vi "CAVRO PUMPS.vi"(0 "Serial Port":refnum<visa-resource-name>="COM3") -> ()   [LabVIEW 2020]
doc: "The Advanced Serial Read and Write example performs a Serial Port Read, a Serial Port Write, or a combination of these actions while setting some advanced serial features like buffer size, termination characters, and XON/XOFF flow control. The user selects the actions (read or write) on the front panel. If both are selected, the VI will write the data first, read the data and then close the VISA session that is opened to the port. \n\nThe parameters set for the serial port must match the parameters of the connected instrument or device. In this example, the bytes to read parameter specifies the number of bytes that the serial port reads. If there were more bytes at the port than the number specified in bytes to read, those bytes would not be read. Also, if you specify to read more bytes than the number of bytes actually read, you might receive a timeout error message.\n\nINSTRUCTIONS:\n1) Select the serial resource and configuration parameters (baud rate, data bits, parity, stop bits, flow control).\n2) Termination character can be enabled and set. Also, set the required input buffer size prior to running the example.\n3) Select the operations to be performed. \n4) Connect the serial port to your device. If no device is available, perform a loopback test by doing one of the following. Short pins 2 and 3 on a RS-232 cable or short pin 4 to pin 8 and pin 5 to pin 9 on a RS-485/422 cable. \n5) Run the VI to see the data read. (The \"read string\" will match the \"string to write\" if a loopback test was performed.)\n\nThis example exposes several advanced features that you may need for your application. Not all applications need all the features shown in this example. The input buffer size is likely an important setting that you want to control in your application. This example expands upon the flow control option for XON and XOFF, allowing the user to choose those control characters. The timeout parameter has been brought to the front panel so a user can specify the time period the VISA Read will wait for the number of bytes to read before timing out. Also, the user has several controls for the termination character, which is discussed later.\n\nNote that you can press the write and read buttons and change the bytes to read parameters on the fly, while the example is running. However, you must stop the example to change the other configuration parameters after the example has started running, and then run again.\n\nSet the I/O buffer size slightly higher the amount of data you expect to receive. This is very important for applications that don't use flow control, as you may lose characters if the receive buffer overflows.\n\nSetting the timeout period ensures that the operation returns with a timeout error if the operation cannot be performed in the specified time period. \n\nSome devices require a termination character in order to identify the end of command strings. Some devices send a termination character to signify the end of data to be read. \n\nThis example shows how you can end the Read operation once a termination character is detected in the buffer and/or append a termination character at the end of the Write data. To enable the Read to end on a termination character, use the VISA Configure Serial Port or use the VISA Properties Serial End Mode for Reads, Termination Character Enable, and Termination Character. To end the Write with a termination character, use the VISA Properties Serial End Mode for Writes, the Send End Enable, and Termination Character. In this example, the same termination character is used for both the Read and the Write. You can specify two different characters for your application, if desired.\n\nYour application may require specific characters for the XON/XOFF Flow Control. You can specify these characters with the VISA Properties Flow Control XOFF Character and Flow Control XON Character. Note that if the standard XON and XOFF characters are used, then decimal 17 and 19 are unavailable for data values. Remember that using flow control and setting an adequate buffer size allow you to prevent buffer overflows."
uses:
  <vilib>/Instr/_visa.llb/VISA Configure Serial Port (Instr).vi
panel:
  in  "Channel":string
  in  "String 3":string
  in  "String 2":string
  in  "String":string="T"
  out "Read buffer":string
  out "Method New/Load":dbl
  in  "WRITE":bool=TRUE
  out "Boolean 2":bool
  out "Boolean":bool
  in  "SLOW SPEED":bool
  in  "FREE COMMAND":bool
  out "String loaded":string caption="String loaded:"
  in  "Load from":path=path "C:/write-read example.txt"
  in  "?":bool
  in  "stop saving":bool
  in  "save":bool
  in  "Save to":path
  in  "INITIALIZE":bool
  in  "END SEQUENCE":bool
  in  "?":string
  in  "DELAY [min]:":bool
  in  "?":string
  in  "GO TO CH:":bool
  in  "INFUSE [uL]:":bool
  out "Command sequence":string
  in  "?":string
  in  "REPEATS & END CICLE":bool
  in  "START CICLE":bool
  in  "REFILL [uL]:":bool
  out "String":string
  in  "START":bool
  # "CAVRO PUMP CONTROLLER"
  # "Load sequence >"
  # "< New sequence"
  # "\"T\" to kill process"
  # "Save to"
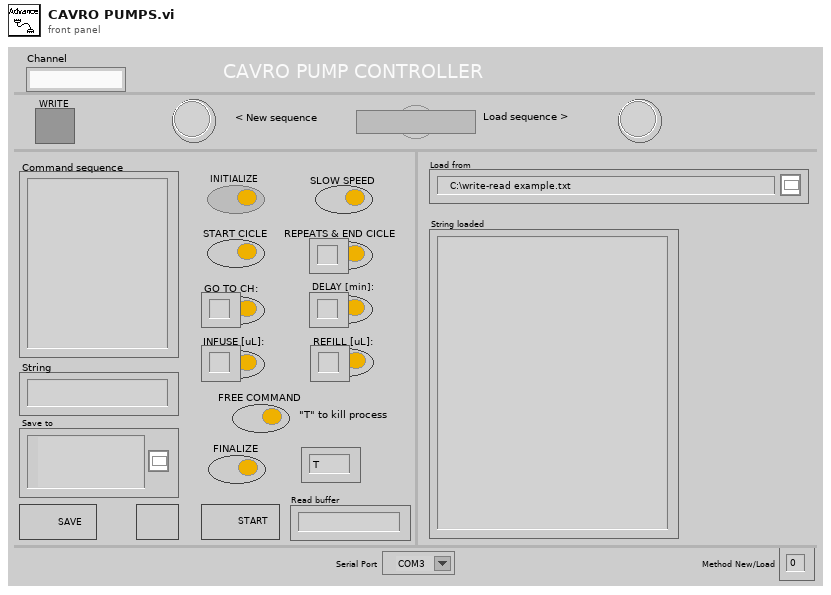
[diagram p1: front panel]
types:
  T1 = enum16{"open", "open or create", "create or replace", "create", "open (read only)"}
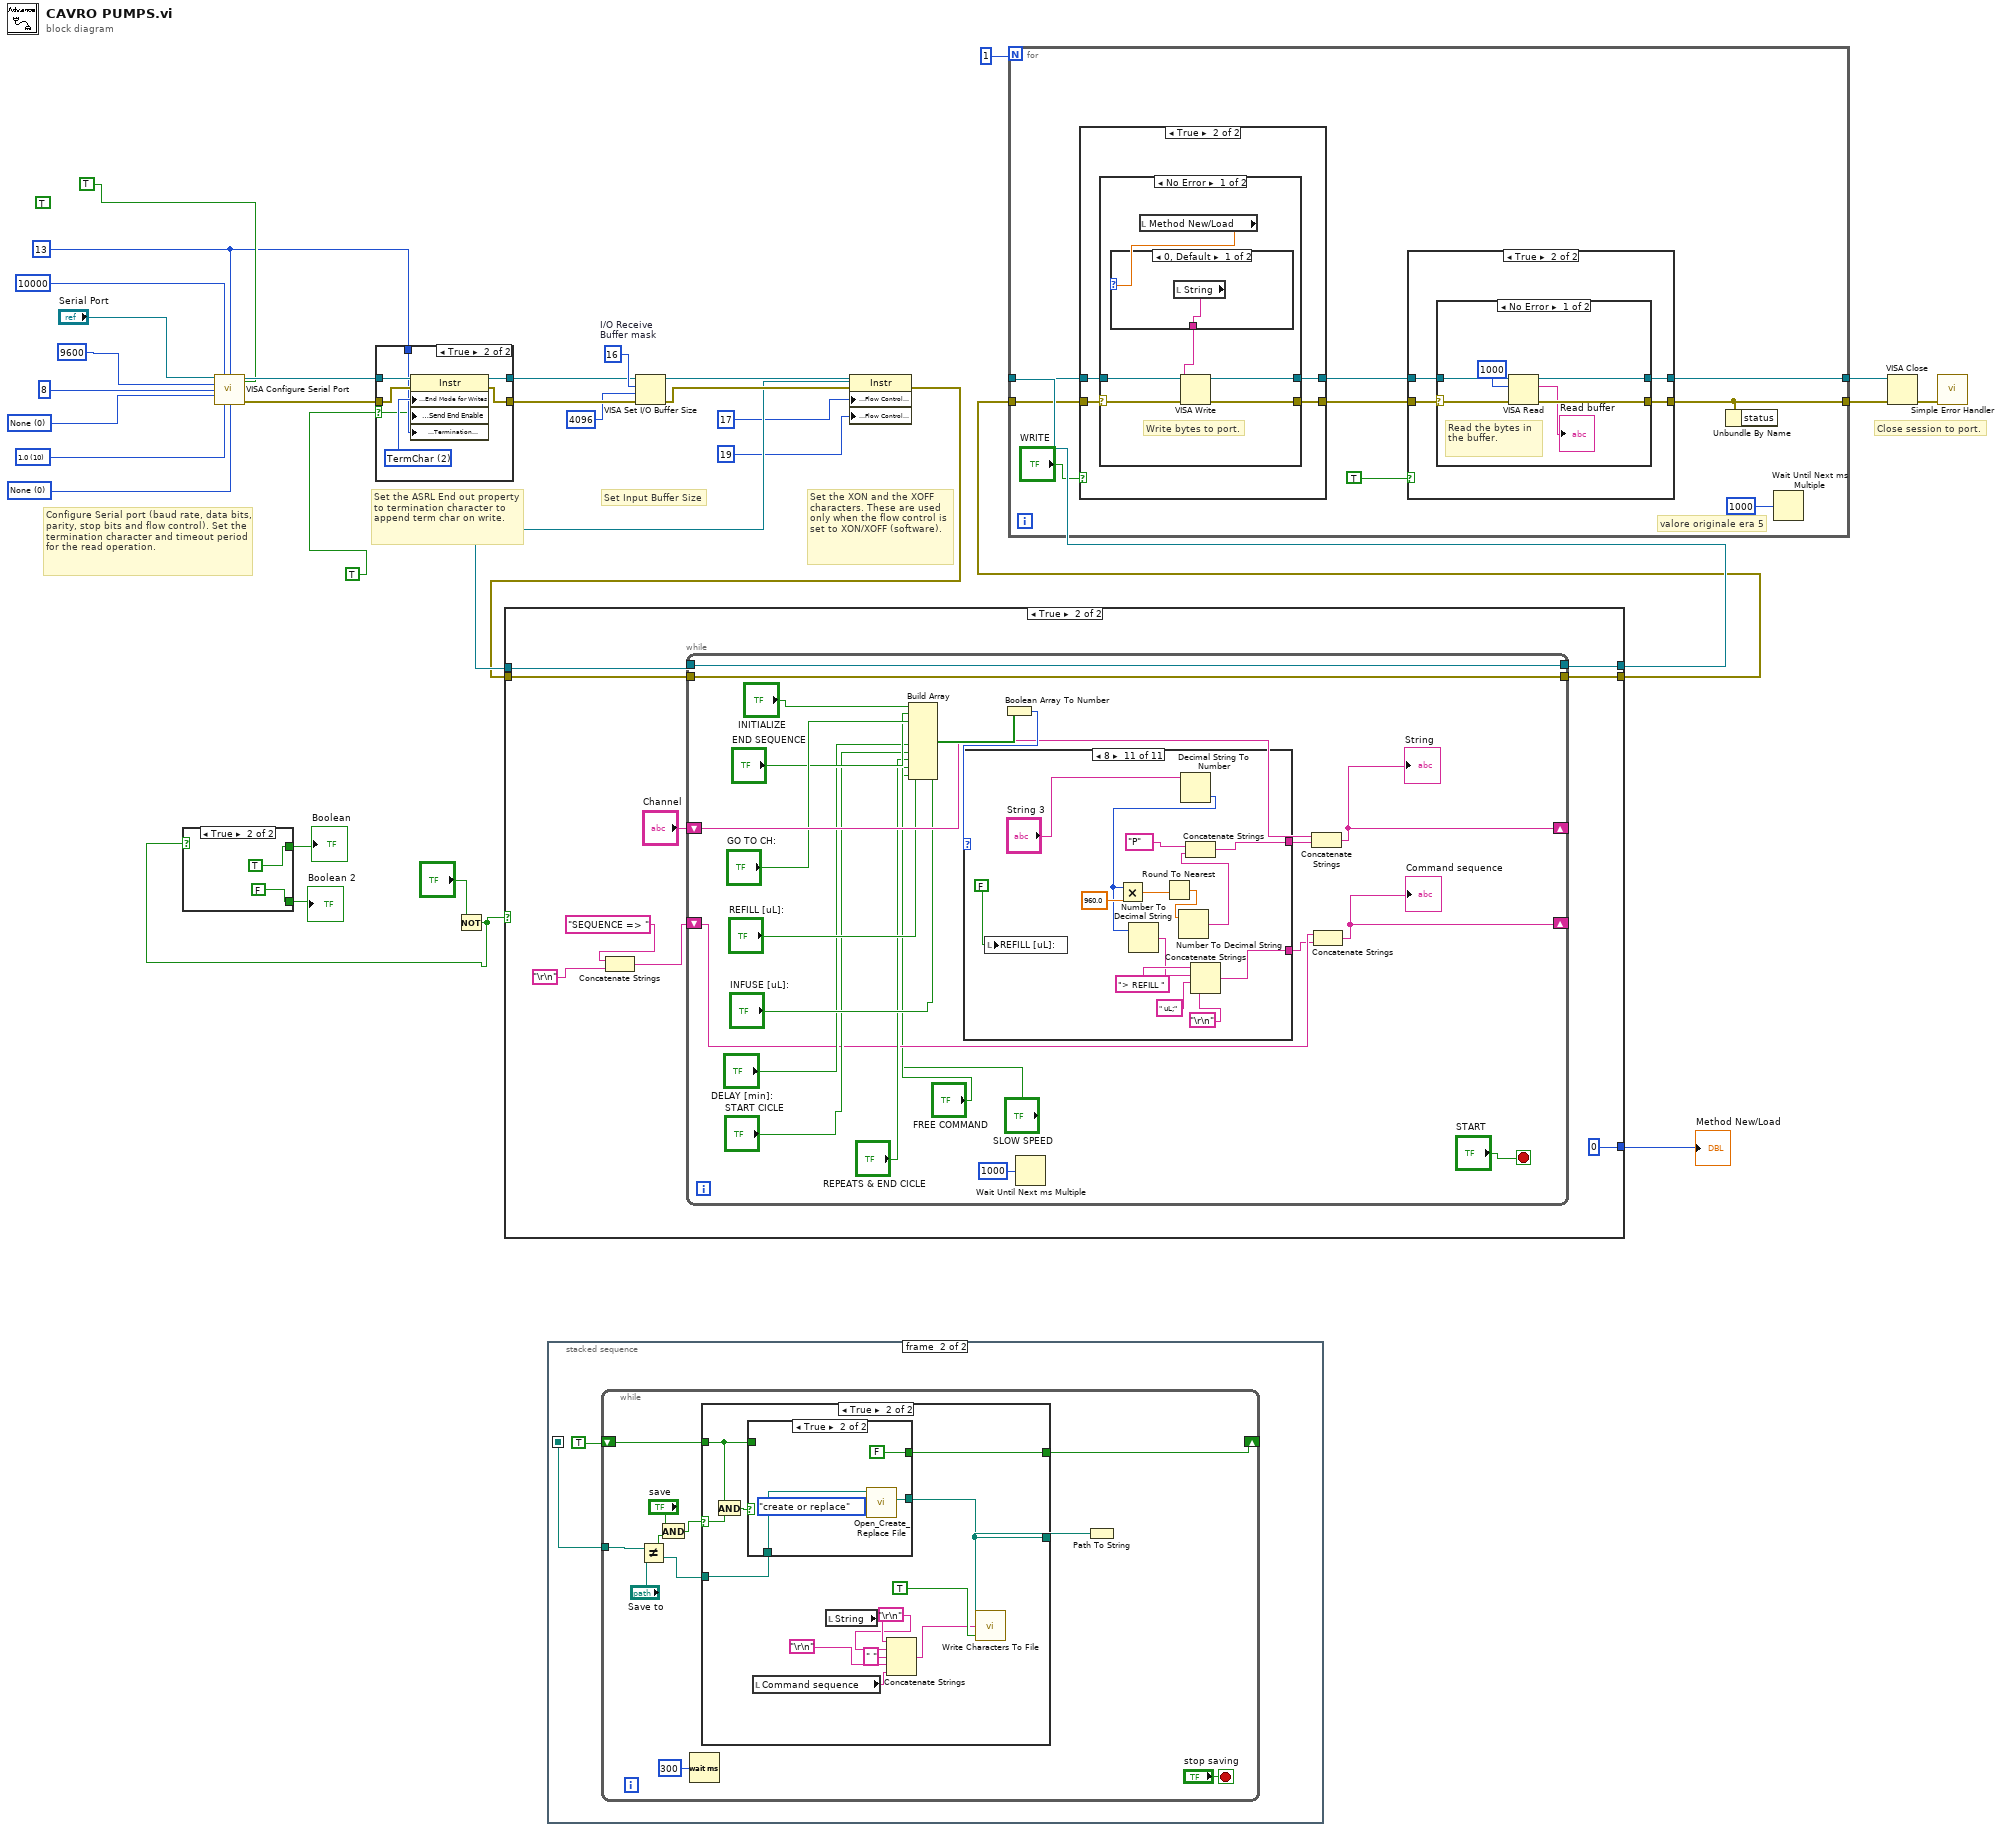
[diagram p0: block diagram]
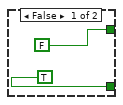
[diagram p2: hidden frame]
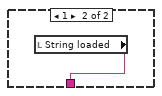
[diagram p4: hidden frame]
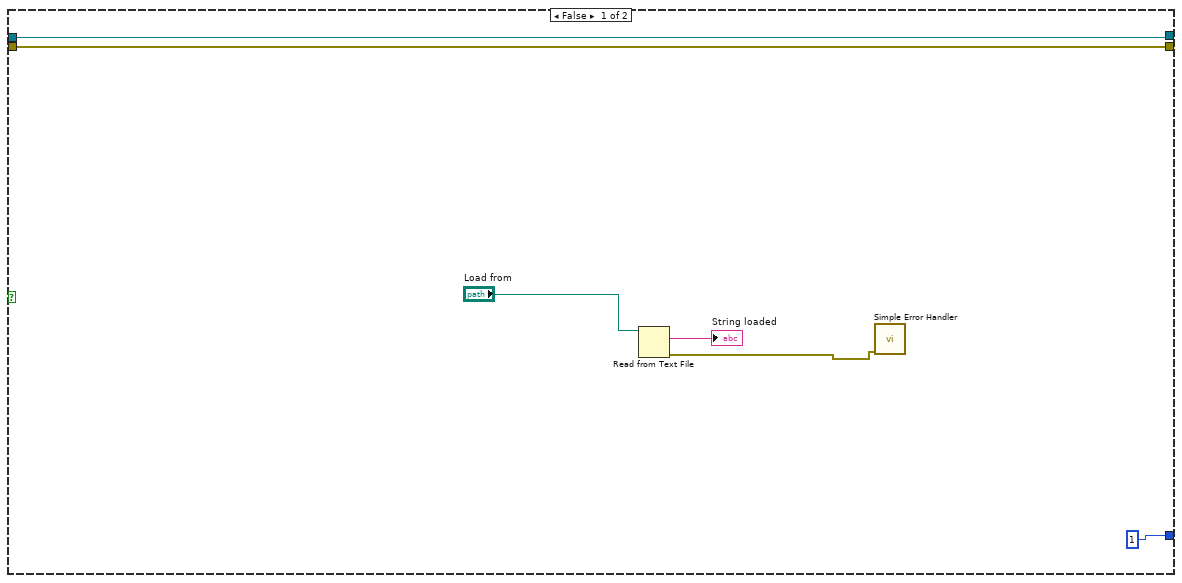
[diagram p8: hidden frame]
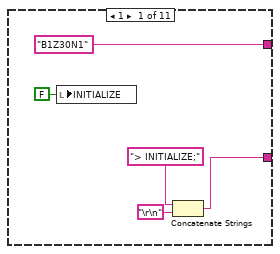
[diagram p9: hidden frame]
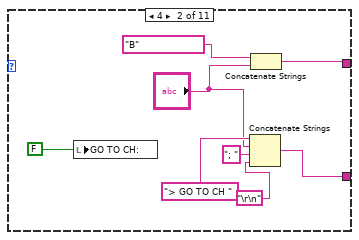
[diagram p10: hidden frame]
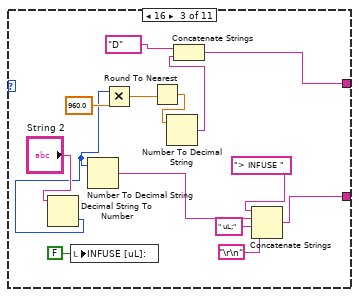
[diagram p11: hidden frame]
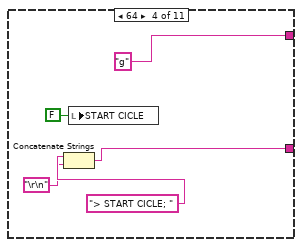
[diagram p12: hidden frame]
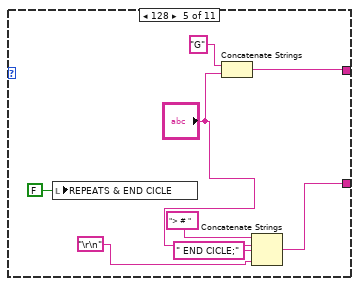
[diagram p13: hidden frame]
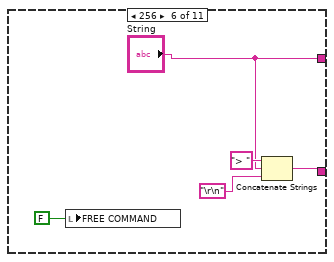
[diagram p14: hidden frame]
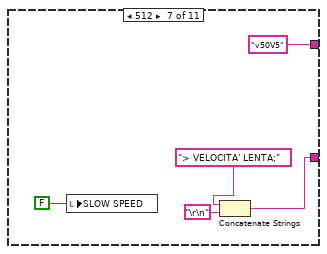
[diagram p15: hidden frame]
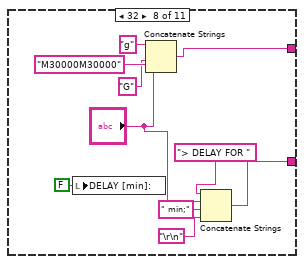
[diagram p16: hidden frame]
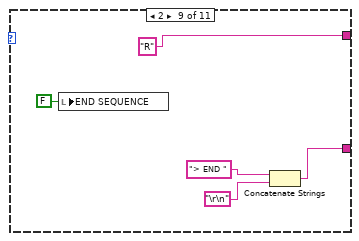
[diagram p17: hidden frame]
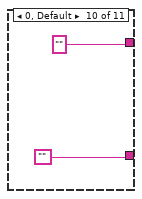
[diagram p18: hidden frame]
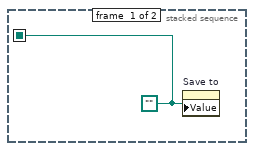
[diagram p19: hidden frame]
diagram:
  w9 = u8 13 ("termination char\n(0xA = '\\n' = LF)")
  w10 = u16 0 items=["None"=0, "XON/XOFF"=1, "RTS/CTS"=2, "DTR/DSR"=4] ("flow control")
  w11 = u16 10 items=["1.0"=10, "1.5"=15, "2.0"=20] ("stop bits")
  w12 = u16 0 items=["None", "Odd", "Even", "Mark", "Space"] ("parity")
  (unwired) TRUE ("End read on termination character?")
  w31 = u16 16  # I/O Receive Buffer mask
  # "Set the XON and the XOFF characters. These are used only when the flow control is set to XON/XOFF (software)."
  # "Configure Serial port (baud rate, data bits, parity, stop bits and flow control). Set the termination character and timeout period for the read operation."
  # "Set Input Buffer Size"
  # "Set the ASRL End out property to termination character to append term char on write."
  # "Close session to port."
  n1 = call-poly "VISA Configure Serial Port"("VISA resource name"="Serial Port", "timeout (10sec)"=u32 10000 ("timeout (ms)"), "termination char\n(0xA = '\\n' = LF)"=w9, "Enable Termination\nChar (T)"=TRUE ("Enable Termination\nChar (T)"), "baud rate (9600)"=u32 9600, "data bits (8)"=u16 8 ("data bits"), "parity (0:none)"=w12, "stop bits (10: 1 bit)"=w11, "flow control (0:none)"=w10) -> ("VISA resource name out"=w25:refnum<visa-resource-name>, "error out"=w28:errorcluster)  [unwired: 1 in, 4 out]
  n2 = case shown="True" TRUE {
    selector: TRUE -> [_ w36]
    tunnel: w25 -> [w34 w42]
    tunnel: w28 -> [w35 w41]
    tunnel: [w34 w40] -> w26
    tunnel: [w35 w39] -> w27
    tunnel: w9 -> [_ w37]
    frame False {
    }
    frame True {
      w38 = u16 2 items=["None", "LastBit", "TermChar", "Break"] ("Serial Settings:Serial End Mode for Writes")
      n3 = property class="Instr"(reference=w42, error in=w41, "Serial Settings:End Mode for Writes"=w38, "Message Based Settings:Send End Enable"=w36, "Message Based Settings:Termination Character"=w37) -> (reference out=w40:refnum<visa-resource-name>, error out=w39:errorcluster)
    }
  }
  n4 = Not(x="?") -> (.not. x?=w1:bool)
  n5 = case shown="True" w1 {
    tunnel: [FALSE ("Boolean") TRUE ("Boolean")] -> w3
    tunnel: [TRUE ("Boolean 2") FALSE ("Boolean 2")] -> w4
    frame False {
    }
    frame True {
    }
  }
  "Boolean" <- w3
  "Boolean 2" <- w4
  n6 = stacked-sequence {
    seq-local: [w47 _] -> [_ w49]
    frame #0 {
      w47 = path ""
      n7 = property on="Save to" class="Path"("Value"=w47) -> ()  [unwired: 2 in, 2 out]
    }
    frame #1 {
      n8 = while {
        tunnel: w49 -> [w54]
        shift-right: [w50] -> _
        shift-left: TRUE -> [w51]
        stop <- "stop saving" stop-if-true
        n9 = Not Equal?(x=w54, y="Save to") -> (x != y?=w57:bool)
        n10 = And(x="save", y=w57) -> (x .and. y?=w55:bool)
        n11 = Wait (ms)(milliseconds to wait=u32 300) -> ()  [unwired: 1 out]
        n12 = case shown="True" w55 {
          selector: w55 -> [_ w72]
          tunnel: [w61 w70] -> w52
          tunnel: "Save to" -> [w61 w71]
          tunnel: w51 -> [w60 w68]
          tunnel: [w60 w69] -> w50
          frame False {
          }
          frame True {
            n13 = And(x=w68, y=w72) -> (x .and. y?=w73:bool)
            n14 = case shown="True" w73 {
              tunnel: w71 -> [w76 w77]
              tunnel: [w76 w79] -> w70
              tunnel: [w75 FALSE] -> w69
              tunnel: w68 -> [w75 _]
              frame False {
              }
              frame True {
                n15 = call <vilib>:"Open_Create_Replace File.vi"("function (open:0)"=T1."create or replace", "file path"=w77) -> ("new file path"=w79:path)  [unwired: 6 in, 3 out]
              }
            }
            n16 = local read "Command sequence"() -> (w63:string)
            n17 = local read "String"() -> (w66:string)
            n18 = Concatenate Strings(w66, "\r\n", " " ("string"), "\r\n", w63) -> (w67:string)
            n19 = call <vilib>:"Write Characters To File.vi"("append to file? (new file:F)"=TRUE, "character string"=w67, "file path (dialog if empty)"=w70) -> ()  [unwired: 2 in, 1 out]
          }
        }
        n20 = Path To String(path=w52) -> ()  [unwired: 1 out]
      }
    }
  }
  n21 = VISA Set I/O Buffer Size(VISA resource name=w26, mask (16)=w31, size (4096)=u32 4096 ("Input\nbuffer size"), error in (no error)=w27) -> (VISA resource name out=w30:refnum<visa-resource-name>, error out=w29:errorcluster)
  n22 = property class="Instr"(reference=w30, error in=w29, "Serial Settings:Flow Control XON Character"=u8 17 ("XON Character"), "Serial Settings:Flow Control XOFF Character"=u8 19 ("XOFF Character")) -> (reference out=w22:refnum<visa-resource-name>, error out=w21:errorcluster)
  n23 = case shown="True" w1 {
    tunnel: w22 -> [w86 w95]
    tunnel: w21 -> [w85 w94]
    tunnel: [w86 w93] -> w20
    tunnel: [w85 w92] -> w19
    tunnel: [1 0] -> w18
    frame False {
      n24 = Read from Text File(file (use dialog)="Load from") -> (text=→"String loaded":string, error out=w81:errorcluster)  [unwired: 3 in, 2 out]
      n25 = call <vilib>:"Simple Error Handler.vi"("error in (no error)"=w81) -> ()  [unwired: 4 in, 5 out]
    }
    frame True {
      n26 = Concatenate Strings("SEQUENCE => ", "\r\n" ("string")) -> (w90:string)
      n27 = while {
        shift-right: [w113] -> _
        shift-left: "Channel" -> [w112]
        tunnel: w95 -> [w111]
        tunnel: [w111] -> w93
        tunnel: w94 -> [w110]
        tunnel: [w110] -> w92
        shift-right: [w101] -> _
        shift-left: w90 -> [w100]
        stop <- "START" stop-if-true
        n28 = Build Array("INITIALIZE", "END SEQUENCE", "GO TO CH:", "REFILL [uL]:", "INFUSE [uL]:", "DELAY [min]:", "START CICLE", "REPEATS & END CICLE", "FREE COMMAND", "SLOW SPEED") -> (w116:bool[])
        n29 = Boolean Array To Number(Boolean array=w116) -> (number=w115:u32)
        n30 = case shown="8" w115 {
          tunnel: ["B1Z30N1" w129 w139 "g" w157 "String" "v50V5" ("String") w173 "R" "" ("String") w198] -> w114
          tunnel: [w120 w126 w137 w147 w154 w161 w165 w169 w180 "" w188] -> w96
          frame 1 {
            n31 = local write "INITIALIZE"(FALSE ("Boolean 2")) -> ()
            n32 = Concatenate Strings("> INITIALIZE;", "\r\n" ("string")) -> (w120:string)
          }
          frame 4 {
            n33 = local write "GO TO CH:"(FALSE ("VAI AL CANALE:")) -> ()
            n34 = Concatenate Strings("> GO TO CH ", "?", "; " ("string"), "\r\n" ("string")) -> (w126:string)
            n35 = Concatenate Strings("B", "?") -> (w129:string)
          }
          frame 16 {
            n36 = Decimal String To Number(string="String 2") -> (number=w132:i32)  [unwired: 2 in, 1 out]
            n37 = local write "INFUSE [uL]:"(FALSE ("INFUSE [uL]:")) -> ()
            n38 = Number To Decimal String(number=w132) -> (decimal integer string=w134:string)  [unwired: 1 in]
            n39 = Multiply(x=w132, y=960.0) -> (x*y=w142:dbl)
            n40 = Round To Nearest(number=w142) -> (nearest integer value=w141:dbl)
            n41 = Number To Decimal String(number=w141) -> (decimal integer string=w140:string)  [unwired: 1 in]
            n42 = Concatenate Strings("D", w140) -> (w139:string)
            n43 = Concatenate Strings("> INFUSE ", w134, " uL;" ("string"), "\r\n" ("string")) -> (w137:string)
          }
          frame 64 {
            n44 = Concatenate Strings("> START CICLE; ", "\r\n" ("string")) -> (w147:string)
            n45 = local write "START CICLE"(FALSE ("START CICLE")) -> ()
          }
          frame 128 {
            n46 = local write "REPEATS & END CICLE"(FALSE ("END CICLE! REPEAT FOR:")) -> ()
            n47 = Concatenate Strings("G" ("string"), "?") -> (w157:string)
            n48 = Concatenate Strings("> # ", "?", " END CICLE;" ("string"), "\r\n") -> (w154:string)
          }
          frame 256 {
            n49 = local write "FREE COMMAND"(FALSE ("COMANDO GENERICO")) -> ()
            n50 = Concatenate Strings("> " ("string"), "String", "\r\n") -> (w161:string)
          }
          frame 512 {
            n51 = local write "SLOW SPEED"(FALSE ("VELOCITA' LENTA")) -> ()
            n52 = Concatenate Strings("> VELOCITA' LENTA;", "\r\n" ("string")) -> (w165:string)
          }
          frame 32 {
            n53 = local write "DELAY [min]:"(FALSE ("DELAY [min]")) -> ()
            n54 = Concatenate Strings("g" ("string"), "M30000M30000" ("string"), "G" ("string"), "?") -> (w173:string)
            n55 = Concatenate Strings("> DELAY FOR ", "?", " min;" ("string"), "\r\n") -> (w169:string)
          }
          frame 2 {
            n56 = local write "END SEQUENCE"(FALSE ("Boolean 3")) -> ()
            n57 = Concatenate Strings("> END ", "\r\n") -> (w180:string)
          }
          frame 0, Default {
          }
          frame 8 {
            n58 = local write "REFILL [uL]:"(FALSE ("ASPIRA")) -> ()
            n59 = Decimal String To Number(string="String 3") -> (number=w186:i32)  [unwired: 2 in, 1 out]
            n60 = Multiply(x=w186, y=960.0) -> (x*y=w191:dbl)
            n61 = Number To Decimal String(number=w186) -> (decimal integer string=w190:string)  [unwired: 1 in]
            n62 = Round To Nearest(number=w191) -> (nearest integer value=w195:dbl)
            n63 = Number To Decimal String(number=w195) -> (decimal integer string=w194:string)  [unwired: 1 in]
            n64 = Concatenate Strings("P", w194) -> (w198:string)
            n65 = Concatenate Strings("> REFILL ", w190, " uL;" ("string"), "\r\n") -> (w188:string)
          }
        }
        n66 = Wait Until Next ms Multiple(millisecond multiple=u32 1000) -> ()  [unwired: 1 out]
        n67 = Concatenate Strings(w112, w114) -> (w113:string)
        "String" <- w113
        n68 = Concatenate Strings(w100, w96) -> (w101:string)
        "Command sequence" <- w101
      }
    }
  }
  "Method New/Load" <- w18
  n69 = for {
    N: 1 -> [_]
    tunnel: w19 -> [w202]
    tunnel: w20 -> [w203]
    tunnel: [w201] -> w24
    tunnel: [w200] -> w23
    # "valore originale era 5"
    n70 = case shown="True" "WRITE" {
      tunnel: [w209 w213] -> w205
      tunnel: [w208 w212] -> w204
      tunnel: w203 -> [w209 w211]
      tunnel: w202 -> [w208 w210]
      frame False {
      }
      frame True {
        n71 = case shown="No Error" w210 {
          selector: w210 -> [w217 w223]
          tunnel: [w215 w222] -> w213
          tunnel: [w219 w223] -> w212
          tunnel: w211 -> [w218 w222]
          frame No Error {
            # "Write bytes to port."
            n72 = local read "Method New/Load"() -> (w214:dbl)
            n73 = case shown="0, Default" w214 {
              tunnel: [w220 w221] -> w216
              frame 0, Default {
                n74 = local read "String"() -> (w220:string)
              }
              frame 1 {
                n75 = local read "String loaded"() -> (w221:string)
              }
            }
            n76 = VISA Write(VISA resource name=w218, write buffer=w216, error in (no error)=w217) -> (VISA resource name out=w215:refnum<visa-resource-name>, error out=w219:errorcluster)  [unwired: 1 out]
          }
          frame Error {
          }
        }
      }
    }
    n77 = case shown="True" TRUE ("read") {
      tunnel: w204 -> [w224 w227]
      tunnel: w205 -> [w225 w226]
      tunnel: [w224 w229] -> w200
      tunnel: [w225 w228] -> w201
      frame False {
      }
      frame True {
        n78 = case "Read bytes from port." shown="No Error" w227 {
          selector: w227 -> [w231 w236]
          tunnel: [w234 w236] -> w229
          tunnel: [w235 w237] -> w228
          tunnel: w226 -> [w232 w237]
          frame No Error {
            # "Read the bytes in the buffer."
            n79 = VISA Read(VISA resource name=w232, byte count=u32 1000 ("bytes to read"), error in (no error)=w231) -> (VISA resource name out=w235:refnum<visa-resource-name>, read buffer=→"Read buffer":string, error out=w234:errorcluster)  [unwired: 1 out]
          }
          frame Error {
            # "Error occurred \nreading Bytes at \nSerial Port"
          }
        }
      }
    }
    n80 = Unbundle By Name(w200) -> ()  [unwired: 1 out]
    n81 = Wait Until Next ms Multiple(millisecond multiple=u32 1000) -> ()  [unwired: 1 out]
  }
  n82 = VISA Close(VISA resource name=w24, error in (no error)=w23) -> (error out=w32:errorcluster)
  n83 = call <vilib>:"Simple Error Handler.vi"("error in (no error)"=w32) -> ()  [unwired: 1 in, 8 out]
